vi "Relay - filtered tap.vi"(8 "error in (no error)":errorcluster) -> (0 "error out":errorcluster)   [LabVIEW 2026, in "Tests.lvlib"]
doc: "Verifies a relay tap with a restrictive filter receives only its subset (SRS-LMBR-023, 026). Registers a queue-mode relay whose filter accepts only WARN and more severe, logs an INFO / WARN / ERROR sweep with the global threshold open, and asserts only WARN and ERROR reach the tap's queue in order while INFO is dropped. Integration tier; runs sequentially.\n\nImplements LMBR-T-045 -> SRS-023, SRS-026. Assert-level IDs: Test-ID-Assert-Checklist.md."
uses:
  Tests.lvlib
  src/TypeDefs/Severity.ctl
  src/TypeDefs/Filter.ctl
  src/TypeDefs/FilterMode.ctl
  <vilib>/addons/_JKI Toolkits/Caraya/classes/Assert/Assert False.vi
  <vilib>/addons/_JKI Toolkits/Caraya/classes/Assert/Assert Equal Value_Variant.vi
  <vilib>/addons/_JKI Toolkits/Caraya/classes/Assert/Assert True.vi
  <vilib>/addons/_JKI Toolkits/Caraya/classes/Test/Test.lvclass
  src/Lumberjack.lvlib
  src/Public/Logger.lvclass/Logger.lvclass
  <vilib>/addons/_JKI Toolkits/Caraya/classes/Assert/Assert.lvclass
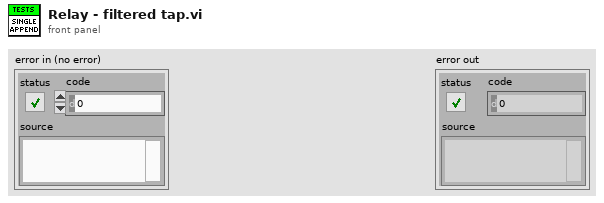
[diagram p1: front panel]
types:
  T1 = typedef "Lumberjack.lvlib/Filter.ctl" = cluster{"mode":T2, "levelMin":T3, "levelMax":T3, "tagPrefix":string}
  T2 = typedef "Lumberjack.lvlib/FilterMode.ctl" = enum16{"Mirror", "Routed"}
  T3 = typedef "Lumberjack.lvlib/Severity.ctl" = enum16{"OFF", "FATAL", "ERROR", "WARN", "INFO", "DEBUG", "TRACE", "ALL"}
  T4 = typedef "Lumberjack.lvlib/Statement.ctl" = cluster{"timestamp":timestamp, "level":T3, "sourceTag":string, "originVI":string, "message":string}
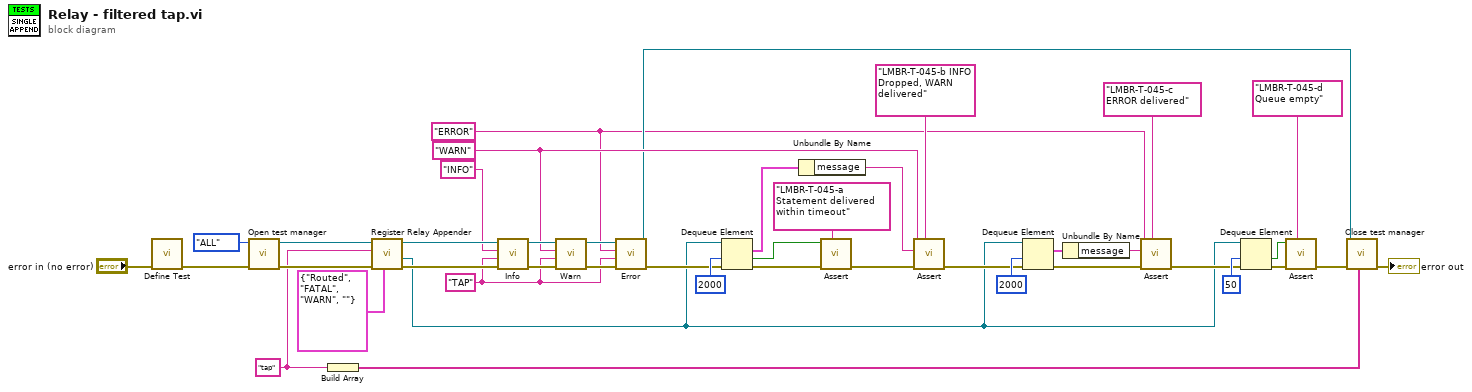
[diagram p0: block diagram]
diagram:
  w13 = "ERROR" ("message")
  w16 = "WARN" ("message")
  w18 = "TAP" ("sourceTag")
  w28 = "tap" ("id in")
  n1 = call <vilib>:"Define Test.vi"("error in (no error)"="error in (no error)") -> ("error out"=w41:errorcluster)  [unwired: 9 in, 1 out]
  n2 = call "Open test manager.vi"("error in (no error)"=w41, "globalThreshold"=Severity."ALL") -> ("error out"=w29:errorcluster, "Logger out"=w30:refnum<class "Logger.lvclass">)  [unwired: 8 in]
  n3 = Build Array(w28) -> (w27:string[])
  n4 = call "Register Relay Appender.vi"("filter"=T1 {"mode"=enum."Routed", "levelMin"=enum."FATAL", "levelMax"=enum."WARN", "tagPrefix"=""}, "error in (no error)"=w29, "id in"=w28, "Logger in"=w30) -> ("error out"=w24:errorcluster, "relayQueue"=w5:refnum<queue>, "Logger out"=w25:refnum<class "Logger.lvclass">)  [unwired: 4 in, 1 out]
  n5 = call "Info.vi"("error in (no error)"=w24, "sourceTag"=w18, "message"="INFO", "Logger in"=w25) -> ("error out"=w22:errorcluster, "Logger out"=w21:refnum<class "Logger.lvclass">)  [unwired: 6 in]
  n6 = call "Warn.vi"("error in (no error)"=w22, "sourceTag"=w18, "message"=w16, "Logger in"=w21) -> ("error out"=w20:errorcluster, "Logger out"=w19:refnum<class "Logger.lvclass">)  [unwired: 6 in]
  n7 = call "Error.vi"("error in (no error)"=w20, "sourceTag"=w18, "message"=w13, "Logger in"=w19) -> ("error out"=w17:errorcluster, "Logger out"=w15:refnum<class "Logger.lvclass">)  [unwired: 6 in]
  n8 = Dequeue Element(queue=w5, timeout in ms (-1)=2000, error in (no error)=w17) -> (element=w35:T4, timed out?=w37:bool, error out=w38:errorcluster)  [unwired: 1 out]
  n9 = Unbundle By Name(w35) -> ("message"=w34:string)
  n10 = call-poly <vilib>:"Assert.vi"("Label"="LMBR-T-045-a Statement delivered within timeout", "error in (no error)"=w38, "False?"=w37) -> ("error out"=w36:errorcluster)  [unwired: 7 in, 1 out]
  n11 = call-poly <vilib>:"Assert.vi"("Label"="LMBR-T-045-b INFO Dropped, WARN delivered", "error in (no error)"=w36, "Actual"=w34, "Expected"=w16) -> ("error out"=w11:errorcluster)  [unwired: 6 in, 1 out]
  n12 = Dequeue Element(queue=w5, timeout in ms (-1)=2000, error in (no error)=w11) -> (element=w9:T4, error out=w10:errorcluster)  [unwired: 2 out]
  n13 = Unbundle By Name(w9) -> ("message"=w8:string)
  n14 = call-poly <vilib>:"Assert.vi"("Label"="LMBR-T-045-c ERROR delivered", "error in (no error)"=w10, "Actual"=w8, "Expected"=w13) -> ("error out"=w6:errorcluster)  [unwired: 6 in, 1 out]
  n15 = Dequeue Element(queue=w5, timeout in ms (-1)=50, error in (no error)=w6) -> (timed out?=w3:bool, error out=w2:errorcluster)  [unwired: 2 out]
  n16 = call-poly <vilib>:"Assert.vi"("Label"="LMBR-T-045-d Queue empty", "error in (no error)"=w2, "True?"=w3) -> ("error out"=w1:errorcluster)  [unwired: 7 in, 1 out]
  n17 = call "Close test manager.vi"("queueIDList"=w27, "error in (no error)"=w1, "Logger in"=w15) -> ("error out"=→"error out":errorcluster)  [unwired: 6 in]
